vi "SerialPort.Write.vi"(8 "error in (no error)":errorcluster, 10 "Data":string, 11 "SerialPort in":refnum<class "SerialPort.lvclass">) -> (0 "error out":errorcluster, 1 "Made Connection":bool, 2 "State":T1, 3 "SerialPort out":refnum<class "SerialPort.lvclass">)   [LabVIEW 2018, in "SerialPort.lvclass"]
uses:
  SerialPort.lvclass
  Controls/SerialPort.Status Enum.ctl
  SerialPort.lvclass/SerialPort.ctl
  Utils/Errors/Error.Error Code List.ctl
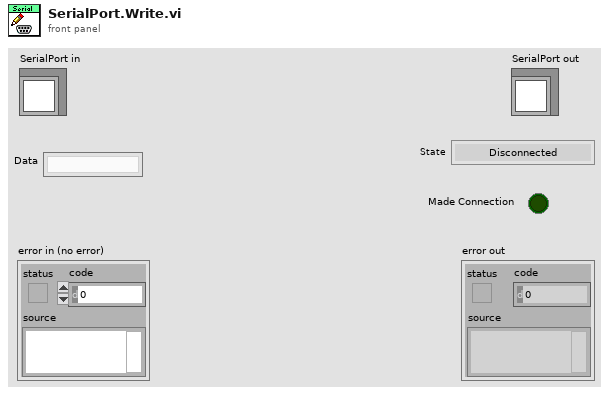
[diagram p1: front panel]
types:
  T1 = typedef "SerialPort.Status Enum.ctl" = enum16{"Disconnected", "Connecting", "Connected"}
  T2 = typedef "Error.Error Code List.ctl" = i32
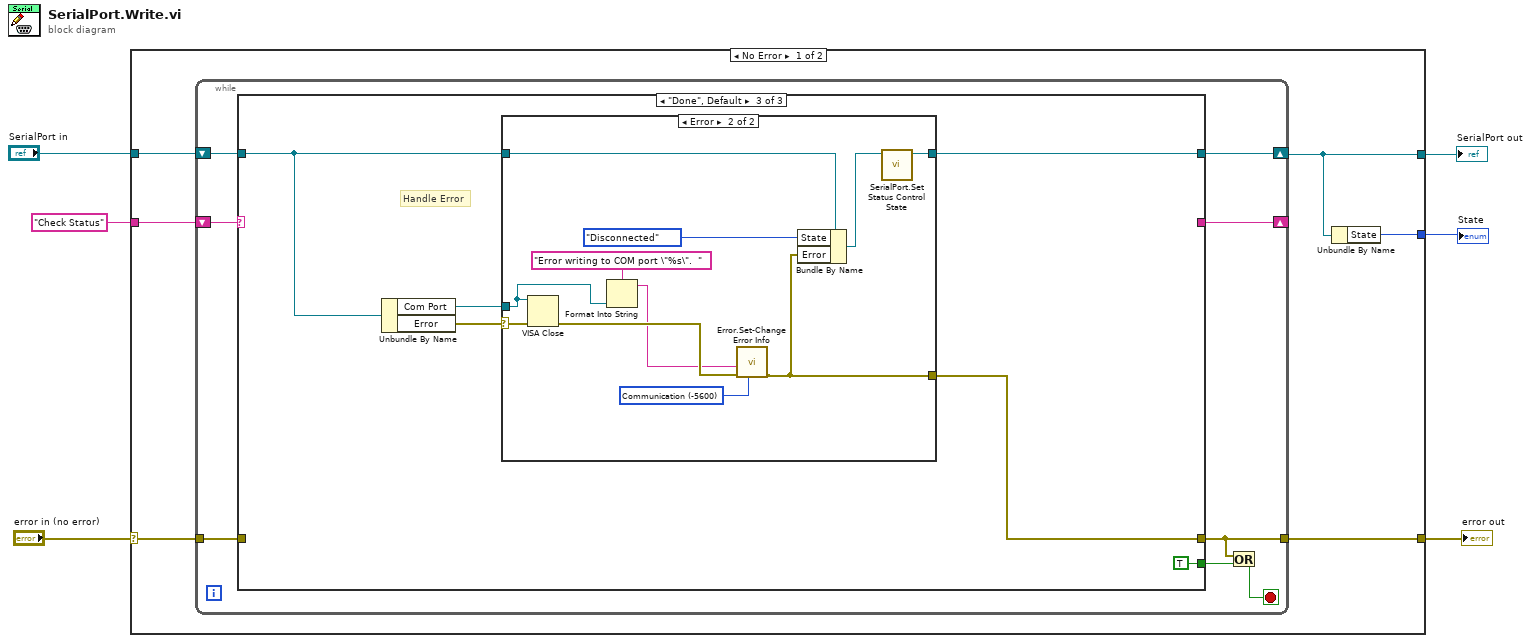
[diagram p0: block diagram]
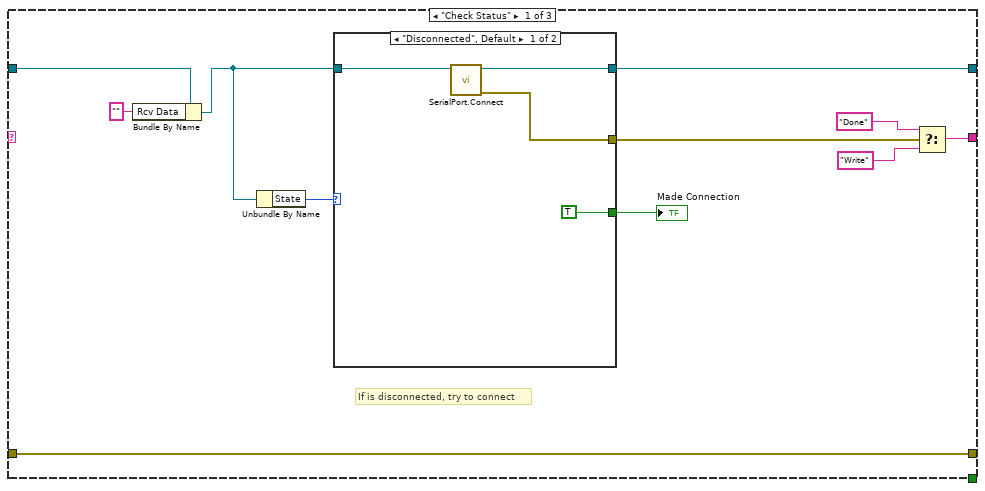
[diagram p2: hidden frame]
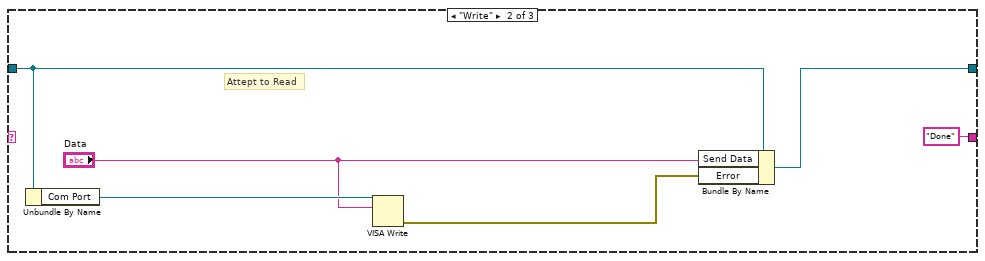
[diagram p4: hidden frame]
diagram:
  n1 = case shown="No Error" "error in (no error)" {
    selector: "error in (no error)" -> [w7 w62]
    tunnel: [w10 w62] -> w5
    tunnel: [w9 w61] -> w3
    tunnel: "SerialPort in" -> [w12 w61]
    tunnel: "Check Status" -> [w11 _]
    tunnel: [w8 _] -> w1
    frame No Error {
      n2 = while {
        shift-right: [w18] -> w9
        shift-left: w12 -> [w19]
        shift-right: [w17] -> _
        shift-left: w11 -> [w20]
        tunnel: [w16] -> w10
        tunnel: w7 -> [w13]
        stop <- w14 stop-if-true
        n3 = case shown="\"Done\", Default" w20 {
          tunnel: w19 -> [w25 w41 w47]
          tunnel: [w30 w40 w43] -> w18
          tunnel: [w29 "Done" _] -> w17
          tunnel: [w22 _ w45] -> w16
          tunnel: [_ _ TRUE] -> w15
          tunnel: w13 -> [w22 _ _]
          frame "Check Status" {
            # "If is disconnected, try to connect"
            n4 = Bundle By Name(cluster=w25, "Rcv Data"="") -> (w24:refnum<class "SerialPort.lvclass">)
            n5 = Unbundle By Name(w24) -> ("State"=w31:T1)
            n6 = case shown="\"Disconnected\", Default" w31 {
              tunnel: w24 -> [w35 w36]
              tunnel: [w34 w36] -> w30
              tunnel: [w33 _] -> w28
              tunnel: [TRUE _] -> w21
              frame "Disconnected", Default {
                n7 = call "SerialPort.Connect.vi"("SerialPort in"=w35) -> ("error out"=w33:errorcluster, "SerialPort out"=w34:refnum<class "SerialPort.lvclass">)  [unwired: 8 in, 1 out]
              }
              frame "Connected" {
              }
            }
            "Made Connection" <- w21
            n8 = Select(t="Done", s=w28, f="Write") -> (s? t:f=w29:string)
          }
          frame "Write" {
            # "Attept to Read"
            n9 = Unbundle By Name(w41) -> ("Com Port"=w39:refnum<visa-resource-name>)
            n10 = VISA Write(VISA resource name=w39, write buffer="Data") -> (error out=w37:errorcluster)  [unwired: 1 in, 2 out]
            n11 = Bundle By Name(cluster=w41, "Send Data"="Data", "Error"=w37) -> (w40:refnum<class "SerialPort.lvclass">)
          }
          frame "Done", Default {
            # "Handle Error"
            n12 = Unbundle By Name(w47) -> ("Com Port"=w46:refnum<visa-resource-name>, "Error"=w48:errorcluster)
            n13 = case shown="Error" w48 {
              selector: w48 -> [w50 w53]
              tunnel: w47 -> [w49 w58]
              tunnel: [w49 w56] -> w43
              tunnel: w46 -> [_ w57]
              tunnel: [w50 w54] -> w45
              frame No Error {
              }
              frame Error {
                w51 = T2 -5600 items=["No Error"=0, "Abort"=-2, "Misc"=-5000, "Fixture Error"=-5100, "File IO - General"=-5200, "FIle IO - Config Error"=-5201, "Instrument - General"=-5300, "Instrument - Serial Com"=-5301, "Instrument - Camera"=-5302, "Instrument - PS"=-5303, "Instrument - Oscilloscope"=-5304, "Instrument - Function Gen"=-5305, "Instrument - Load"=-5306, "Instrument - Meter"=-5307, "Instrument - Power Control"=-5308, "Instrument - Motion"=-5309, "Instrument - RF"=-5310, "System Exe"=-5400, "Image Processing"=-5500, "Communication"=-5600, "Script - Syntax Error"=-6000, "Script - Invalid Name or Param"=-6100, "Script - Timeout"=-6200, "Invalid Data"=-6300] ("Std Code")
                n14 = VISA Close(VISA resource name=w57) -> ()  [unwired: 1 in, 1 out]
                n15 = Format Into String(format string="Error writing to COM port \"%s\".  ", w57) -> (resulting string=w52:string)  [unwired: 2 in, 1 out]
                n16 = call "Error.Set-Change Error Info.vi"("Std Code"=w51, "error in"=w53, "Description"=w52) -> ("error out"=w54:errorcluster)  [unwired: 8 in]
                n17 = Bundle By Name(cluster=w58, "State"=SerialPort.Status_Enum."Disconnected", "Error"=w54) -> (w55:refnum<class "SerialPort.lvclass">)
                n18 = call "SerialPort.Set Status Control State.vi"("SerialPort in"=w55) -> ("SerialPort out"=w56:refnum<class "SerialPort.lvclass">)  [unwired: 9 in, 1 out]
              }
            }
          }
        }
        n19 = Or(x=w16, y=w15) -> (x .or. y?=w14:bool)
      }
      n20 = Unbundle By Name(w9) -> ("State"=w8:T1)
    }
    frame Error {
    }
  }
  "error out" <- w5
  "SerialPort out" <- w3
  "State" <- w1
